vi "List Sessions.vi"(8 "error in (no error)":errorcluster, 11 "CSM-Static-Variable-Manager in":refnum<class "CSM-Static-Variable-Manager.lvclass">) -> (0 "error out":errorcluster, 1 "Array":string[](array[string]), 3 "CSM-Static-Variable-Manager out":refnum<class "CSM-Static-Variable-Manager.lvclass">)   [LabVIEW 2017, in "INI-Static-Variable-Support.lvlib" / "CSM-Static-Variable-Manager.lvclass"]
uses:
  CSM-Static-Variable-Manager.lvclass
  CSM-Static-Variable-Manager.lvclass/CSM-Static-Variable-Manager.ctl
  LabVIEW-Config/LabVIEW-Config.lvclass
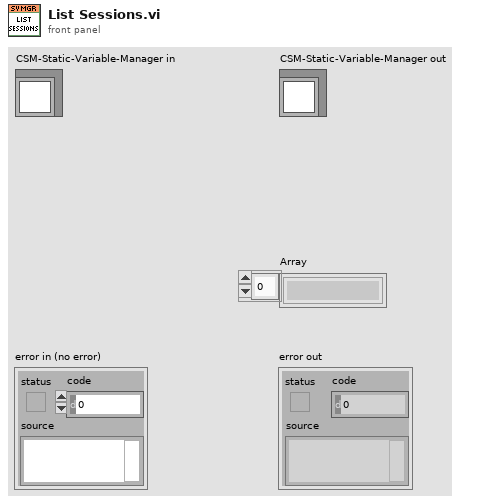
[diagram p1: front panel]
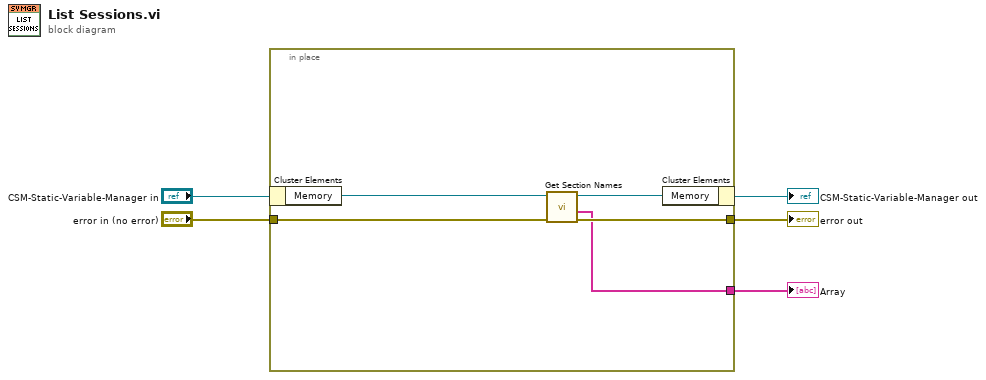
[diagram p0: block diagram]
diagram:
  n1 = in-place {
    in-place-border: "error in (no error)" -> [w8]
    in-place-border: [w7] -> w2
    in-place-border: [w6] -> w1
    n2 = in-place-cluster #1("CSM-Static-Variable-Manager in") -> ("Memory"=w10:refnum<class "LabVIEW-Config.lvclass">)
    n3 = call "Get Section Names.vi"("error in (no error)"=w8, "Config in"=w10) -> ("error out"=w7:errorcluster, "Section Names"=w6:string[], "Config out"=w9:refnum<class "LabVIEW-Config.lvclass">)  [unwired: 7 in]
    n4 = in-place-cluster #1("Memory"=w9) -> (→"CSM-Static-Variable-Manager out":refnum<class "CSM-Static-Variable-Manager.lvclass">)
  }
  "error out" <- w2
  "Array" <- w1
